vi "Read_Wrap_Simple.vi"() -> (1 "Value":T1)   [LabVIEW 2021, in "Var_DBL.lvclass"]
uses:
  Type.ctl
  Var_DBL.lvclass
  Var_DBL.lvclass/Var_DBL.ctl
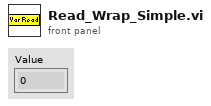
[diagram p1: front panel]
types:
  T1 = typedef "Var_DBL.lvclass/Type.ctl" = dbl
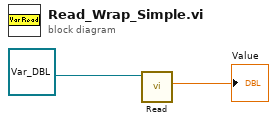
[diagram p0: block diagram]
diagram:
  n1 = call-dynamic "Read.vi"("Numeric in"=refnum<class "Var_DBL.lvclass"> refnum ("Constants.lvlib:Numeric.lvclass")) -> ("Numeric"=→"Value":T1)  [unwired: 8 in, 2 out]
